vi "Query Log.vi"(7 "Project":string, 8 "error in (no error)":errorcluster caption="Error In", 9 "Stop Time":timestamp format="%<%x %.3X>T", 10 "Start Time":timestamp format="%<%x %.3X>T", 11 "Table":string(combo)) -> (0 "error out":errorcluster caption="Error Out", 3 "data":string[][](array[string]))   [LabVIEW 2020]
uses:
  <vilib>/addons/database/_DB Variant To Data/Database Variant To Data.xnode
  <vilib>/addons/database/NI_Database_API.lvlib
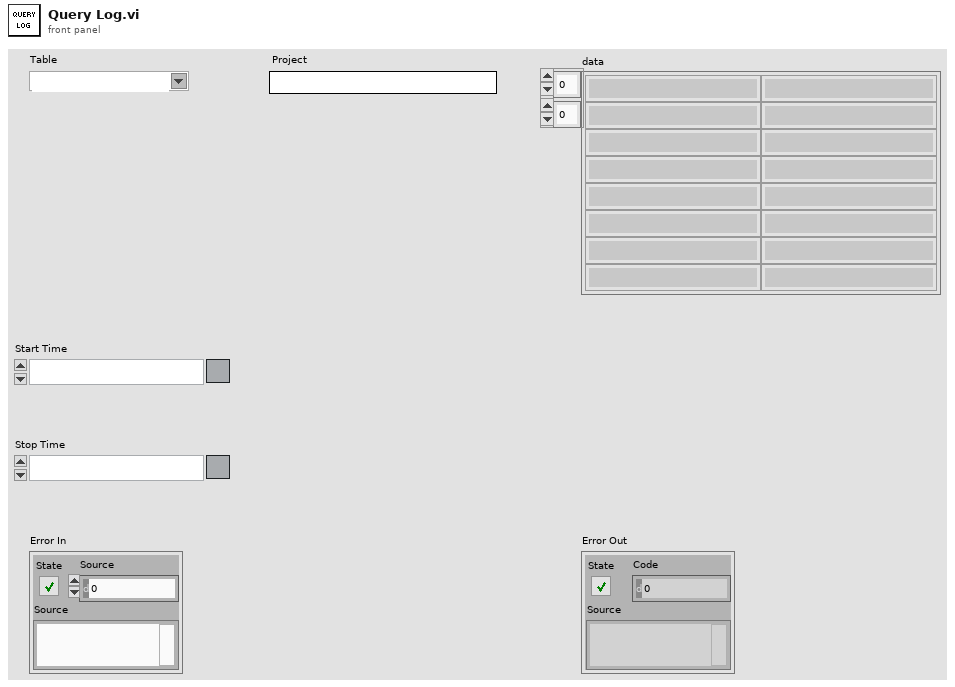
[diagram p1: front panel]
types:
  T1 = typedef "NI_Database_API.lvlib/Conn ObjectReference.ctl" = refnum<k1>
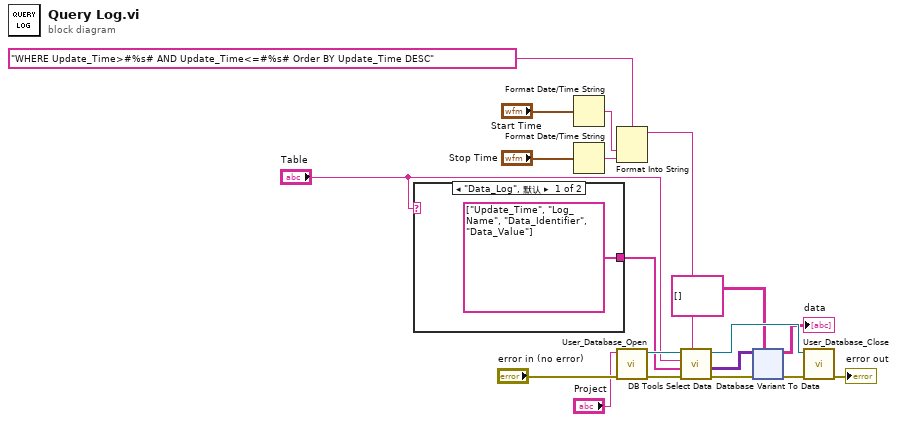
[diagram p0: block diagram]
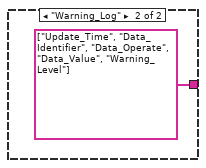
[diagram p2: hidden frame]
diagram:
  n1 = case shown="\"Data_Log\", 默认" "Table" {
    tunnel: [string[] ["Update_Time", "Log_Name", "Data_Identifier", "Data_Value"] string[] ["Update_Time", "Data_Identifier", "Data_Operate", "Data_Value", "Warning_Level"]] -> w2
    frame "Data_Log", Default {
    }
    frame "Warning_Log" {
    }
  }
  n2 = Format Date/Time String(seconds (now)="Start Time") -> (date/time string=w6:string)  [unwired: 2 in]
  n3 = Format Date/Time String(seconds (now)="Stop Time") -> (date/time string=w5:string)  [unwired: 2 in]
  n4 = Format Into String(format string="WHERE Update_Time>#%s# AND Update_Time<=#%s# Order BY Update_Time DESC" ("格式字符串"), w6, w5) -> (resulting string=w4:string)  [unwired: 2 in, 1 out]
  n5 = call "User_Database_Open.vi"("error in (no error)"="error in (no error)", "Project"="Project") -> ("error out"=w16:errorcluster, "DB Ref Out"=w17:T1)  [unwired: 8 in]
  n6 = call <vilib>:"DB Tools Select Data.vi"("condition"=w4, "error in (no error)"=w16, "columns"=w2, "table"="Table", "connection reference"=w17) -> ("error out"=w15:errorcluster, "data"=w11:variant[][], "connection reference out"=w14:T1)  [unwired: 1 in]
  n7 = xnode "Database Variant To Data"("database variant"=w11, "error in (no error)"=w15, "type"=string[][] []) -> ("data"=→"data":string[][], "error out"=w13:errorcluster)
  n8 = call "User_Database_Close.vi"("error in (no error)"=w13, "DB Ref In"=w14) -> ("error out"=→"error out":errorcluster)  [unwired: 9 in]
